vi "Ball Shooter Delay.vi"(8 "Ball Release \nDelay in Milliseconds":i32=3000, 9 "Delay after Ball is Release":u32=500, 10 "Delay in Milliseconds":i32=3000, 11 "Shoot ball":bool) -> (0 "Total Number of shots made":i16, 2 "Ball Release":bool, 3 "Shooter Motor":bool)   [LabVIEW 2012]
panel:
  # "1000 Milliseconds = 1 Second"
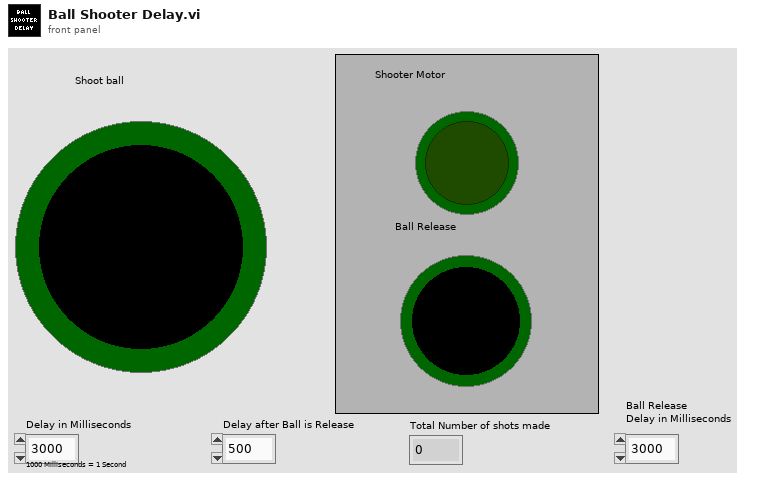
[diagram p1: front panel]
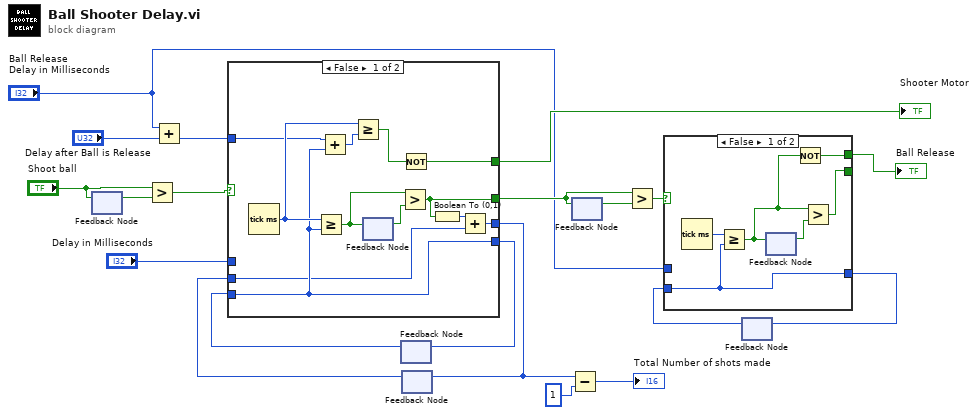
[diagram p0: block diagram]
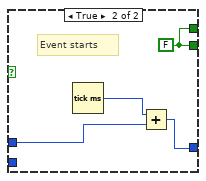
[diagram p2: hidden frame]
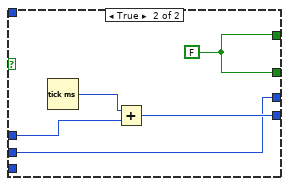
[diagram p3: hidden frame]
diagram:
  n1 = feedback #1() -> (w16:bool)  [unwired: 1 in]
  n2 = feedback-in #1("Shoot ball") -> ()
  n3 = Greater?(x="Shoot ball", y=w16) -> (0:w17:bool)
  n4 = Add(x="Ball Release \nDelay in Milliseconds", y="Delay after Ball is Release") -> (x+y=w2:u32)
  n5 = feedback #2() -> (w20:u32)  [unwired: 1 in]
  n6 = feedback #3() -> (w13:i16)  [unwired: 1 in]
  n7 = case shown="False" w17 {
    tunnel: "Delay in Milliseconds" -> [_ w35]
    tunnel: [w27 w36] -> w19
    tunnel: [w25 w34] -> w6
    tunnel: w20 -> [w27 _]
    tunnel: [w30 w34] -> w14
    tunnel: [w23 w33] -> w11
    tunnel: w13 -> [w22 w33]
    tunnel: w2 -> [w21 _]
    frame False {
      n8 = Tick Count (ms)() -> (millisecond timer value=w29:u32)
      n9 = Greater Or Equal?(x=w29, y=w27) -> (x >= y?=w31:bool)
      n10 = Add(x=w21, y=w27) -> (x+y=w28:u32)
      n11 = Greater Or Equal?(x=w29, y=w28) -> (x >= y?=w26:bool)
      n12 = feedback #4() -> (w32:bool)  [unwired: 1 in]
      n13 = feedback-in #4(w31) -> ()
      n14 = Greater?(x=w31, y=w32) -> (0:w25:bool)
      n15 = Not(x=w26) -> (.not. x?=w30:bool)
      n16 = Boolean To (0,1)(Boolean=w25) -> (0, 1=w24:i16)
      n17 = Add(x=w24, y=w22) -> (x+y=w23:i16)
    }
    frame True {
      w34 = FALSE
      n18 = Tick Count (ms)() -> (millisecond timer value=w37:u32)
      n19 = Add(x=w37, y=w35) -> (x+y=w36:u32)
    }
  }
  "Shooter Motor" <- w14
  n20 = feedback-in #2(w19) -> ()
  n21 = feedback-in #3(w11) -> ()
  n22 = Subtract(x=w11, y=i16 1 ("x")) -> (x-y=→"Total Number of shots made":i16)
  n23 = feedback #5() -> (w8:bool)  [unwired: 1 in]
  n24 = feedback-in #5(w6) -> ()
  n25 = Greater?(x=w6, y=w8) -> (0:w7:bool)
  n26 = feedback #6() -> (w4:u32)  [unwired: 1 in]
  n27 = case shown="False" w7 {
    tunnel: "Ball Release \nDelay in Milliseconds" -> [_ w45]
    tunnel: [w41 w46] -> w5
    tunnel: w4 -> [w41 _]
    tunnel: [w40 w44] -> _
    tunnel: [w38 w44] -> w3
    frame False {
      n28 = Tick Count (ms)() -> (millisecond timer value=w43:u32)
      n29 = Greater Or Equal?(x=w43, y=w41) -> (x >= y?=w39:bool)
      n30 = feedback #7() -> (w42:bool)  [unwired: 1 in]
      n31 = feedback-in #7(w39) -> ()
      n32 = Not(x=w39) -> (.not. x?=w38:bool)
      n33 = Greater?(x=w39, y=w42) -> (0:w40:bool)
    }
    frame True {
      w44 = FALSE
      # "Event starts"
      n34 = Tick Count (ms)() -> (millisecond timer value=w47:u32)
      n35 = Add(x=w47, y=w45) -> (x+y=w46:u32)
    }
  }
  "Ball Release" <- w3
  n36 = feedback-in #6(w5) -> ()
